vi "Get CPU ID.vi"() -> ()   [LabVIEW 2013, in "ManagementClass.lvclass"]
uses:
  ManagementClass.lvclass
panel:
  out "Processor ID":string="512"
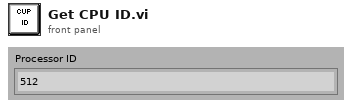
[diagram p1: front panel]
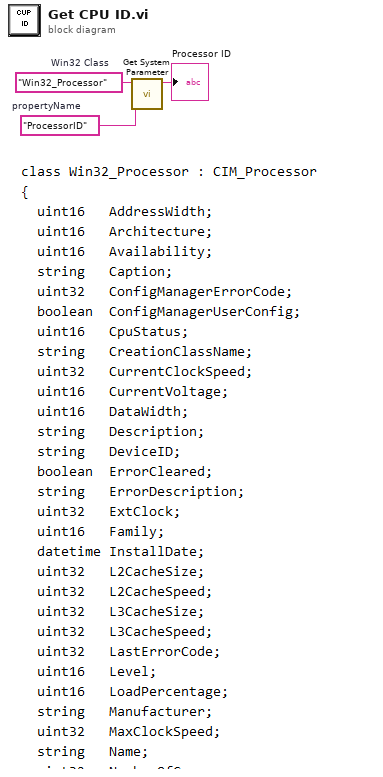
[diagram p0: block diagram]
diagram:
  w1 = "ProcessorID"  # propertyName
  w2 = "Win32_Processor"  # Win32 Class
  n1 = call "Get System Parameter.vi"("propertyName"=w1, "path"=w2) -> ("propertyValue"=→"Processor ID":string)  [unwired: 8 in, 1 out]
